vi "ble_search_client_characteristic_conf_handle.vi"(8 "error in (no error)":errorcluster, 9 "Characteristic UUID":string, 10 "Service UUID":string, 11 "Handle table":string[][](array[string])) -> (0 "error out":errorcluster, 2 "Handle":string)   [LabVIEW 2013]
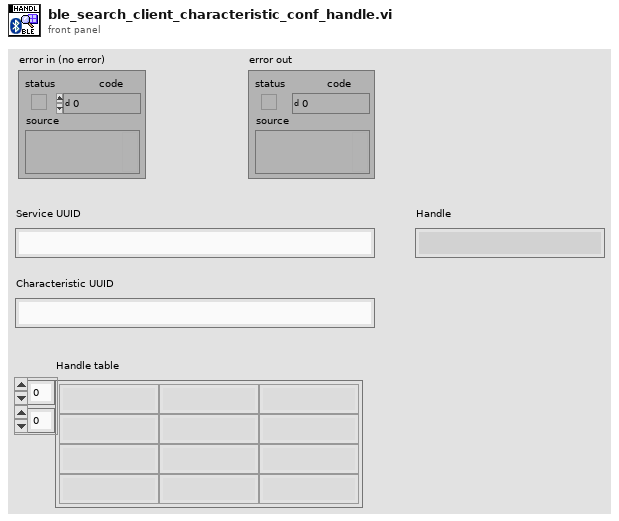
[diagram p1: front panel]
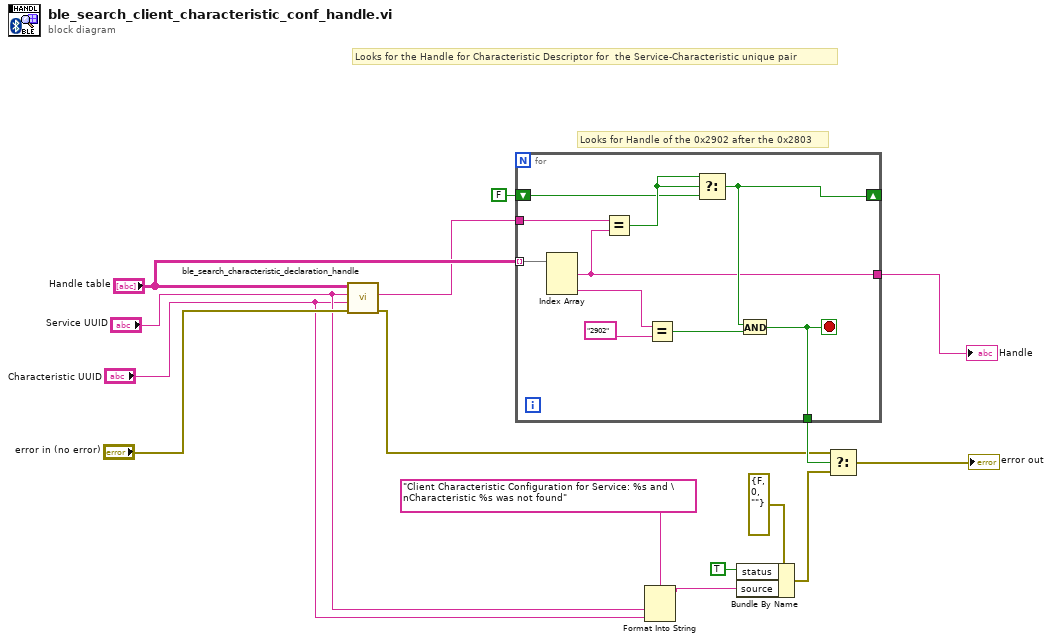
[diagram p0: block diagram]
diagram:
  # "Looks for Handle of the 0x2902 after the 0x2803"
  # "Looks for the Handle for Characteristic Descriptor for  the Service-Characteristic unique pair"
  n1 = call "ble_search_characteristic_declaration_handle.vi"("error in (no error)"="error in (no error)", "Characteristic UUID"="Characteristic UUID", "Service UUID"="Service UUID", "Handle table"="Handle table") -> ("error out"=w7:errorcluster, "Handle"=w3:string)  [unwired: 6 in]
  n2 = for {
    tunnel: "Handle table" -> [w25] mode=indexing
    tunnel: w3 -> [w24]
    tunnel: [w16] -> w9
    shift-right: [w19] -> _
    shift-left: FALSE -> [w20]
    tunnel: [w17] -> w1
    stop <- w16 stop-if-true
    n3 = Index Array(array=w25) -> (element #1=w17:string, element #3=w22:string)  [unwired: 3 in, 1 out]
    n4 = Equal?(x=w24, y=w17) -> (x = y?=w21:bool)
    n5 = Equal?(x=w22, y="2902") -> (x = y?=w18:bool)
    n6 = Select(t=w21, s=w21, f=w20) -> (s? t:f=w19:bool)
    n7 = And(x=w19, y=w18) -> (x .and. y?=w16:bool)
  }
  "Handle" <- w1
  n8 = Format Into String(format string="Client Characteristic Configuration for Service: %s and \nCharacteristic %s was not found", "Service UUID", "Characteristic UUID") -> (resulting string=w10:string)  [unwired: 2 in, 1 out]
  n9 = Bundle By Name(cluster=errorcluster {"status"=FALSE, "code"=0, "source"=""} ("error in (no error)"), "status"=TRUE, "source"=w10) -> (w14:errorcluster)
  n10 = Select(t=w7, s=w9, f=w14) -> (s? t:f=→"error out":errorcluster)
